vi "GPM DB Connection String--constant.vi"() -> (3 "DB Connection String":string)   [LabVIEW 2016, in "Packages.lvlib" / "GPM.lvlib"]
uses:
  GPM.lvlib
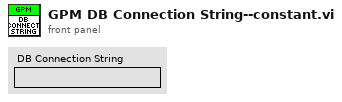
[diagram p1: front panel]
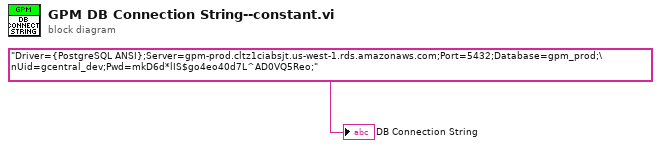
[diagram p0: block diagram]
diagram:
  "DB Connection String" <- "Driver={PostgreSQL ANSI};Server=gpm-prod.cltz1ciabsjt.us-west-1.rds.amazonaws.com;Port=5432;Database=gpm_prod;\nUid=gcentral_dev;Pwd=mkD6d*lIS$go4eo40d7L^AD0VQ5Reo;"
